vi "GeoData.vi"() -> ()   [LabVIEW 2017] (continued)
TN\tWeakley County\tH1\n38230\t47183\tGreenfield\tTN\tWeakley County\tH1\n38229\t47183\tGleason\tTN\tWeakley County\tH1\n38238\t47183\tMartin\tTN\tWeakley County\tH1\n38261\t47183\tUnion city\tTN\tWeakley County\tH1\n38224\t47183\tCottage grove\tTN\tWeakley County\tH1\n38257\t47183\tSouth fulton\tTN\tWeakley County\tH1\n38241\t47183\tPalmersville\tTN\tWeakley County\tH1\n38506\t47185\tCookeville\tTN\tWhite County\tH1\n38583\t47185\tSparta\tTN\tWhite County\tH1\n38579\t47185\tQuebeck\tTN\tWhite County\tH1\n38587\t47185\tWalling\tTN\tWhite County\tH1\n38559\t47185\tDoyle\tTN\tWhite County\tH1\n37060\t47187\tEagleville\tTN\tWilliamson County\tH1\n37211\t47187\tNashville\tTN\tWilliamson County\tH1\n37179\t47187\tThompsons station\tTN\tWilliamson County\tH1\n37062\t47187\tFairview\tTN\tWilliamson County\tH1\n37215\t47187\tNashville\tTN\tWilliamson County\tH1\n37221\t47187\tNashville\tTN\tWilliamson County\tH1\n37014\t47187\tArrington\tTN\tWilliamson County\tH1\n37174\t47187\tSpring hill\tTN\tWilliamson County\tH1\n37135\t47187\tNolensville\tTN\tWilliamson County\tH1\n37027\t47187\tBrentwood\tTN\tWilliamson County\tH1\n37067\t47187\tFranklin\tTN\tWilliamson County\tH1\n37082\t47187\tKingston springs\tTN\tWilliamson County\tH1\n37046\t47187\tCollege grove\tTN\tWilliamson County\tH1\n37064\t47187\tFranklin\tTN\tWilliamson County\tH1\n38401\t47187\tColumbia\tTN\tWilliamson County\tH1\n37069\t47187\tFranklin\tTN\tWilliamson County\tH1\n37065\t47187\tFranklin\tTN\tWilliamson County\tH1\n38476\t47187\tPrimm springs\tTN\tWilliamson County\tH1\n37025\t47187\tBon aqua\tTN\tWilliamson County\tH1\n37068\t47187\tFranklin\tTN\tWilliamson County\tH1\n37118\t47189\tMilton\tTN\tWilson County\tH1\n37076\t47189\tHermitage\tTN\tWilson County\tH1\n37016\t47189\tAuburntown\tTN\tWilson County\tH1\n37090\t47189\tLebanon\tTN\tWilson County\tH1\n37122\t47189\tMount juliet\tTN\tWilson County\tH1\n37138\t47189\tOld hickory\tTN\tWilson County\tH1\n37095\t47189\tLiberty\tTN\tWilson County\tH1\n37121\t47189\tMount juliet\tTN\tWilson County\tH1\n37012\t47189\tAlexandria\tTN\tWilson County\tH1\n37184\t47189\tWatertown\tTN\tWilson County\tH1\n37088\t47189\tLebanon\tTN\tWilson County\tH1\n37087\t47189\tLebanon\tTN\tWilson County\tH1\n37085\t47189\tLascassas\tTN\tWilson County\tH1\n37071\t47189\tGladeville\tTN\tWilson County\tH1\n75779\t48001\tNeches\tTX\tAnderson County\tH1\n75803\t48001\tPalestine\tTX\tAnderson County\tH1\n75763\t48001\tFrankston\tTX\tAnderson County\tH1\n75844\t48001\tGrapeland\tTX\tAnderson County\tH1\n75751\t48001\tAthens\tTX\tAnderson County\tH1\n75884\t48001\tTennessee colony\tTX\tAnderson County\tH1\n75853\t48001\tMontalba\tTX\tAnderson County\tH1\n75832\t48001\tCayuga\tTX\tAnderson County\tH1\n75861\t48001\tTennessee colony\tTX\tAnderson County\tH1\n75882\t48001\tPalestine\tTX\tAnderson County\tH1\n75839\t48001\tElkhart\tTX\tAnderson County\tH1\n75880\t48001\tTennessee colony\tTX\tAnderson County\tH1\n75801\t48001\tPalestine\tTX\tAnderson County\tH1\n75752\t48001\tAthens\tTX\tAnderson County\tH1\n75770\t48001\tLarue\tTX\tAnderson County\tH1\n75802\t48001\tPalestine\tTX\tAnderson County\tH1\n75886\t48001\tTennessee colony\tTX\tAnderson County\tH1\n79714\t48003\tAndrews\tTX\tAndrews County\tH1\n75915\t48005\tLufkin\tTX\tAngelina County\tH1\n75901\t48005\tLufkin\tTX\tAngelina County\tH1\n75902\t48005\tLufkin\tTX\tAngelina County\tH1\n75949\t48005\tHuntington\tTX\tAngelina County\tH1\n75951\t48005\tJasper\tTX\tAngelina County\tH1\n75980\t48005\tZavalla\tTX\tAngelina County\tH1\n75941\t48005\tDiboll\tTX\tAngelina County\tH1\n75903\t48005\tLufkin\tTX\tAngelina County\tH1\n75904\t48005\tLufkin\tTX\tAngelina County\tH1\n75969\t48005\tPollok\tTX\tAngelina County\tH1\n78382\t48007\tRockport\tTX\tAransas County\tH1\n78390\t48007\tTaft\tTX\tAransas County\tH1\n78381\t48007\tRockport\tTX\tAransas County\tH1\n78336\t48007\tAransas pass\tTX\tAransas County\tH1\n78358\t48007\tFulton\tTX\tAransas County\tH1\n76360\t48009\tElectra\tTX\tArcher County\tH1\n76310\t48009\tWichita falls\tTX\tArcher County\tH1\n76302\t48009\tWichita falls\tTX\tArcher County\tH1\n76374\t48009\tOlney\tTX\tArcher County\tH1\n76366\t48009\tHolliday\tTX\tArcher County\tH1\n76379\t48009\tScotland\tTX\tArcher County\tH1\n76389\t48009\tWindthorst\tTX\tArcher County\tH1\n76370\t48009\tMegargel\tTX\tArcher County\tH1\n76308\t48009\tWichita falls\tTX\tArcher County\tH1\n76351\t48009\tArcher city\tTX\tArcher County\tH1\n79226\t48011\tClarendon\tTX\tArmstrong County\tH1\n79039\t48011\tGroom\tTX\tArmstrong County\tH1\n79042\t48011\tHappy\tTX\tArmstrong County\tH1\n79118\t48011\tAmarillo\tTX\tArmstrong County\tH1\n79019\t48011\tClaude\tTX\tArmstrong County\tH1\n79094\t48011\tWayside\tTX\tArmstrong County\tH1\n78113\t48013\tFalls city\tTX\tAtascosa County\tH1\n78011\t48013\tCharlotte\tTX\tAtascosa County\tH1\n78012\t48013\tChristine\tTX\tAtascosa County\tH1\n78114\t48013\tFloresville\tTX\tAtascosa County\tH1\n78064\t48013\tPleasanton\tTX\tAtascosa County\tH1\n78118\t48013\tKarnes city\tTX\tAtascosa County\tH1\n78052\t48013\tLytle\tTX\tAtascosa County\tH1\n78002\t48013\tAtascosa\tTX\tAtascosa County\tH1\n78065\t48013\tPoteet\tTX\tAtascosa County\tH1\n78264\t48013\tSan antonio\tTX\tAtascosa County\tH1\n78069\t48013\tSomerset\tTX\tAtascosa County\tH1\n78050\t48013\tLeming\tTX\tAtascosa County\tH1\n78073\t48013\tVon ormy\tTX\tAtascosa County\tH1\n78008\t48013\tCampbellton\tTX\tAtascosa County\tH1\n78005\t48013\tBigfoot\tTX\tAtascosa County\tH1\n78021\t48013\tFowlerton\tTX\tAtascosa County\tH1\n78026\t48013\tJourdanton\tTX\tAtascosa County\tH1\n77833\t48015\tBrenham\tTX\tAustin County\tH1\n78933\t48015\tCat spring\tTX\tAustin County\tH1\n77474\t48015\tSealy\tTX\tAustin County\tH1\n78940\t48015\tFayetteville\tTX\tAustin County\tH1\n77452\t48015\tKenney\tTX\tAustin County\tH1\n77835\t48015\tBurton\tTX\tAustin County\tH1\n78954\t48015\tRound top\tTX\tAustin County\tH1\n77418\t48015\tBellville\tTX\tAustin County\tH1\n78944\t48015\tIndustry\tTX\tAustin County\tH1\n77473\t48015\tSan felipe\tTX\tAustin County\tH1\n78950\t48015\tNew ulm\tTX\tAustin County\tH1\n77426\t48015\tChappell hill\tTX\tAustin County\tH1\n77485\t48015\tWallis\tTX\tAustin County\tH1\n78931\t48015\tBleiblerville\tTX\tAustin County\tH1\n79324\t48017\tEnochs\tTX\tBailey County\tH1\n79031\t48017\tEarth\tTX\tBailey County\tH1\n79325\t48017\tFarwell\tTX\tBailey County\tH1\n79346\t48017\tMorton\tTX\tBailey County\tH1\n79347\t48017\tMuleshoe\tTX\tBailey County\tH1\n79344\t48017\tMaple\tTX\tBailey County\tH1\n79371\t48017\tSudan\tTX\tBailey County\tH1\n78023\t48019\tHelotes\tTX\tBandera County\tH1\n78055\t48019\tMedina\tTX\tBandera County\tH1\n78010\t48019\tCenter point\tTX\tBandera County\tH1\n78883\t48019\tTarpley\tTX\tBandera County\tH1\n78063\t48019\tPipe creek\tTX\tBandera County\tH1\n78884\t48019\tUtopia\tTX\tBandera County\tH1\n78003\t48019\tBandera\tTX\tBandera County\tH1\n78885\t48019\tVanderpool\tTX\tBandera County\tH1\n78942\t48021\tGiddings\tTX\tBastrop County\tH1\n78959\t48021\tWaelder\tTX\tBastrop County\tH1\n78616\t48021\tDale\tTX\tBastrop County\tH1\n78659\t48021\tPaige\tTX\tBastrop County\tH1\n78612\t48021\tCedar creek\tTX\tBastrop County\tH1\n78941\t48021\tFlatonia\tTX\tBastrop County\tH1\n78953\t48021\tRosanky\tTX\tBastrop County\tH1\n78617\t48021\tDel valle\tTX\tBastrop County\tH1\n78957\t48021\tSmithville\tTX\tBastrop County\tH1\n78650\t48021\tMc dade\tTX\tBastrop County\tH1\n78662\t48021\tRed rock\tTX\tBastrop County\tH1\n78602\t48021\tBastrop\tTX\tBastrop County\tH1\n78621\t48021\tElgin\tTX\tBastrop County\tH1\n78653\t48021\tManor\tTX\tBastrop County\tH1\n76380\t48023\tSeymour\tTX\tBaylor County\tH1\n78391\t48025\tTynan\tTX\tBee County\tH1\n78162\t48025\tTuleta\tTX\tBee County\tH1\n78102\t48025\tBeeville\tTX\tBee County\tH1\n78119\t48025\tKenedy\tTX\tBee County\tH1\n78389\t48025\tSkidmore\tTX\tBee County\tH1\n78071\t48025\tThree rivers\tTX\tBee County\tH1\n78368\t48025\tMathis\tTX\tBee County\tH1\n78125\t48025\tMineral\tTX\tBee County\tH1\n78142\t48025\tNormanna\tTX\tBee County\tH1\n78145\t48025\tPawnee\tTX\tBee County\tH1\n78104\t48025\tBeeville\tTX\tBee County\tH1\n78146\t48025\tPettus\tTX\tBee County\tH1\n78387\t48025\tSinton\tTX\tBee County\tH1\n76541\t48027\tKilleen\tTX\tBell County\tH1\n76569\t48027\tRogers\tTX\tBell County\tH1\n76519\t48027\tBurlington\tTX\tBell County\tH1\n76533\t48027\tHeidenheimer\tTX\tBell County\tH1\n76502\t48027\tTemple\tTX\tBell County\tH1\n76513\t48027\tBelton\tTX\tBell County\tH1\n76579\t48027\tTroy\tTX\tBell County\tH1\n76528\t48027\tGatesville\tTX\tBell County\tH1\n76557\t48027\tMoody\tTX\tBell County\tH1\n76559\t48027\tNolanville\tTX\tBell County\tH1\n76537\t48027\tJarrell\tTX\tBell County\tH1\n76547\t48027\tKilleen\tTX\tBell County\tH1\n76549\t48027\tKilleen\tTX\tBell County\tH1\n76508\t48027\tTemple\tTX\tBell County\tH1\n76542\t48027\tKilleen\tTX\tBell County\tH1\n76548\t48027\tHarker heights\tTX\tBell County\tH1\n76571\t48027\tSalado\tTX\tBell County\tH1\n76527\t48027\tFlorence\tTX\tBell County\tH1\n76570\t48027\tRosebud\tTX\tBell County\tH1\n76504\t48027\tTemple\tTX\tBell County\tH1\n76554\t48027\tLittle river academy\tTX\tBell County\tH1\n76539\t48027\tKempner\tTX\tBell County\tH1\n76540\t48027\tKilleen\tTX\tBell County\tH1\n76501\t48027\tTemple\tTX\tBell County\tH1\n76564\t48027\tPendleton\tTX\tBell County\tH1\n76503\t48027\tTemple\tTX\tBell County\tH1\n76543\t48027\tKilleen\tTX\tBell County\tH1\n76511\t48027\tBartlett\tTX\tBell County\tH1\n76544\t48027\tFort hood\tTX\tBell County\tH1\n76656\t48027\tLott\tTX\tBell County\tH1\n76534\t48027\tHolland\tTX\tBell County\tH1\n78023\t48029\tHelotes\tTX\tBexar County\tH1\n78039\t48029\tLa coste\tTX\tBexar County\tH1\n78210\t48029\tSan antonio\tTX\tBexar County\tH1\n78260\t48029\tSan antonio\tTX\tBexar County\tH1\n78270\t48029\tSan antonio\tTX\tBexar County\tH1\n78239\t48029\tSan antonio\tTX\tBexar County\tH1\n78244\t48029\tSan antonio\tTX\tBexar County\tH1\n78235\t48029\tSan antonio\tTX\tBexar County\tH1\n78288\t48029\tSan antonio\tTX\tBexar County\tH1\n78297\t48029\tSan antonio\tTX\tBexar County\tH1\n78246\t48029\tSan antonio\tTX\tBexar County\tH1\n78124\t48029\tMarion\tTX\tBexar County\tH1\n78214\t48029\tSan antonio\tTX\tBexar County\tH1\n78202\t48029\tSan antonio\tTX\tBexar County\tH1\n78207\t48029\tSan antonio\tTX\tBexar County\tH1\n78222\t48029\tSan antonio\tTX\tBexar County\tH1\n78224\t48029\tSan antonio\tTX\tBexar County\tH1\n78259\t48029\tSan antonio\tTX\tBexar County\tH1\n78150\t48029\tJbsa randolph\tTX\tBexar County\tH1\n78296\t48029\tSan antonio\tTX\tBexar County\tH1\n78291\t48029\tSan antonio\tTX\tBexar County\tH1\n78054\t48029\tMacdona\tTX\tBexar County\tH1\n78148\t48029\tUniversal city\tTX\tBexar County\tH1\n78217\t48029\tSan antonio\tTX\tBexar County\tH1\n78208\t48029\tSan antonio\tTX\tBexar County\tH1\n78215\t48029\tSan antonio\tTX\tBexar County\tH1\n78225\t48029\tSan antonio\tTX\tBexar County\tH1\n78226\t48029\tSan antonio\tTX\tBexar County\tH1\n78250\t48029\tSan antonio\tTX\tBexar County\tH1\n78266\t48029\tSan antonio\tTX\tBexar County\tH1\n78263\t48029\tSan antonio\tTX\tBexar County\tH1\n78206\t48029\tSan antonio\tTX\tBexar County\tH1\n78268\t48029\tSan antonio\tTX\tBexar County\tH1\n78298\t48029\tSan antonio\tTX\tBexar County\tH1\n78294\t48029\tSan antonio\tTX\tBexar County\tH1\n78292\t48029\tSan antonio\tTX\tBexar County\tH1\n78006\t48029\tBoerne\tTX\tBexar County\tH1\n78108\t48029\tCibolo\tTX\tBexar County\tH1\n78052\t48029\tLytle\tTX\tBexar County\tH1\n78212\t48029\tSan antonio\tTX\tBexar County\tH1\n78205\t48029\tSan antonio\tTX\tBexar County\tH1\n78229\t48029\tSan antonio\tTX\tBexar County\tH1\n78233\t48029\tSan antonio\tTX\tBexar County\tH1\n78232\t48029\tSan antonio\tTX\tBexar County\tH1\n78240\t48029\tSan antonio\tTX\tBexar County\tH1\n78237\t48029\tSan antonio\tTX\tBexar County\tH1\n78251\t48029\tSan antonio\tTX\tBexar County\tH1\n78269\t48029\tSan antonio\tTX\tBexar County\tH1\n78002\t48029\tAtascosa\tTX\tBexar County\tH1\n78101\t48029\tAdkins\tTX\tBexar County\tH1\n78209\t48029\tSan antonio\tTX\tBexar County\tH1\n78220\t48029\tSan antonio\tTX\tBexar County\tH1\n78216\t48029\tSan antonio\tTX\tBexar County\tH1\n78163\t48029\tBulverde\tTX\tBexar County\tH1\n78204\t48029\tSan antonio\tTX\tBexar County\tH1\n78231\t48029\tSan antonio\tTX\tBexar County\tH1\n78264\t48029\tSan antonio\tTX\tBexar County\tH1\n78256\t48029\tSan antonio\tTX\tBexar County\tH1\n78234\t48029\tJbsa ft sam houston\tTX\tBexar County\tH1\n78253\t48029\tSan antonio\tTX\tBexar County\tH1\n78254\t48029\tSan antonio\tTX\tBexar County\tH1\n78069\t48029\tSomerset\tTX\tBexar County\tH1\n78299\t48029\tSan antonio\tTX\tBexar County\tH1\n78252\t48029\tSan antonio\tTX\tBexar County\tH1\n78284\t48029\tSan antonio\tTX\tBexar County\tH1\n78285\t48029\tSan antonio\tTX\tBexar County\tH1\n78009\t48029\tCastroville\tTX\tBexar County\tH1\n78073\t48029\tVon ormy\tTX\tBexar County\tH1\n78154\t48029\tSchertz\tTX\tBexar County\tH1\n78221\t48029\tSan antonio\tTX\tBexar County\tH1\n78201\t48029\tSan antonio\tTX\tBexar County\tH1\n78213\t48029\tSan antonio\tTX\tBexar County\tH1\n78228\t48029\tSan antonio\tTX\tBexar County\tH1\n78230\t48029\tSan antonio\tTX\tBexar County\tH1\n78258\t48029\tSan antonio\tTX\tBexar County\tH1\n78245\t48029\tSan antonio\tTX\tBexar County\tH1\n78242\t48029\tSan antonio\tTX\tBexar County\tH1\n78238\t48029\tSan antonio\tTX\tBexar County\tH1\n78295\t48029\tSan antonio\tTX\tBexar County\tH1\n78152\t48029\tSaint hedwig\tTX\tBexar County\tH1\n78243\t48029\tSan antonio\tTX\tBexar County\tH1\n78015\t48029\tBoerne\tTX\tBexar County\tH1\n78109\t48029\tConverse\tTX\tBexar County\tH1\n78112\t48029\tElmendorf\tTX\tBexar County\tH1\n78218\t48029\tSan antonio\tTX\tBexar County\tH1\n78219\t48029\tSan antonio\tTX\tBexar County\tH1\n78223\t48029\tSan antonio\tTX\tBexar County\tH1\n78227\t48029\tSan antonio\tTX\tBexar County\tH1\n78203\t48029\tSan antonio\tTX\tBexar County\tH1\n78247\t48029\tSan antonio\tTX\tBexar County\tH1\n78249\t48029\tSan antonio\tTX\tBexar County\tH1\n78257\t48029\tSan antonio\tTX\tBexar County\tH1\n78283\t48029\tSan antonio\tTX\tBexar County\tH1\n78265\t48029\tSan antonio\tTX\tBexar County\tH1\n78278\t48029\tSan antonio\tTX\tBexar County\tH1\n78293\t48029\tSan antonio\tTX\tBexar County\tH1\n78241\t48029\tSan antonio\tTX\tBexar County\tH1\n78211\t48029\tSan antonio\tTX\tBexar County\tH1\n78248\t48029\tSan antonio\tTX\tBexar County\tH1\n78236\t48029\tJbsa lackland\tTX\tBexar County\tH1\n78255\t48029\tSan antonio\tTX\tBexar County\tH1\n78261\t48029\tSan antonio\tTX\tBexar County\tH1\n78280\t48029\tSan antonio\tTX\tBexar County\tH1\n78279\t48029\tSan antonio\tTX\tBexar County\tH1\n78635\t48031\tHye\tTX\tBlanco County\tH1\n78027\t48031\tKendalia\tTX\tBlanco County\tH1\n78620\t48031\tDripping springs\tTX\tBlanco County\tH1\n78636\t48031\tJohnson city\tTX\tBlanco County\tH1\n78663\t48031\tRound mountain\tTX\tBlanco County\tH1\n78676\t48031\tWimberley\tTX\tBlanco County\tH1\n78070\t48031\tSpring branch\tTX\tBlanco County\tH1\n78669\t48031\tSpicewood\tTX\tBlanco County\tH1\n78671\t48031\tStonewall\tTX\tBlanco County\tH1\n78606\t48031\tBlanco\tTX\tBlanco County\tH1\n79356\t48033\tPost\tTX\tBorden County\tH1\n79713\t48033\tAckerly\tTX\tBorden County\tH1\n79738\t48033\tGail\tTX\tBorden County\tH1\n79511\t48033\tCoahoma\tTX\tBorden County\tH1\n79517\t48033\tFluvanna\tTX\tBorden County\tH1\n79527\t48033\tIra\tTX\tBorden County\tH1\n79351\t48033\tOdonnell\tTX\tBorden County\tH1\n76633\t48035\tChina spring\tTX\tBosque County\tH1\n76043\t48035\tGlen rose\tTX\tBosque County\tH1\n76528\t48035\tGatesville\tTX\tBosque County\tH1\n76652\t48035\tKopperl\tTX\tBosque County\tH1\n76457\t48035\tHico\tTX\tBosque County\tH1\n76634\t48035\tClifton\tTX\tBosque County\tH1\n76665\t48035\tMeridian\tTX\tBosque County\tH1\n76671\t48035\tMorgan\tTX\tBosque County\tH1\n76649\t48035\tIredell\tTX\tBosque County\tH1\n76689\t48035\tValley mills\tTX\tBosque County\tH1\n76690\t48035\tWalnut springs\tTX\tBosque County\tH1\n76637\t48035\tCranfills gap\tTX\tBosque County\tH1\n75501\t48037\tTexarkana\tTX\tBowie County\tH1\n75560\t48037\tDouglassville\tTX\tBowie County\tH1\n75573\t48037\tRedwater\tTX\tBowie County\tH1\n75567\t48037\tMaud\tTX\tBowie County\tH1\n75554\t48037\tAvery\tTX\tBowie County\tH1\n75503\t48037\tTexarkana\tTX\tBowie County\tH1\n75505\t48037\tTexarkana\tTX\tBowie County\tH1\n75570\t48037\tNew boston\tTX\tBowie County\tH1\n75561\t48037\tHooks\tTX\tBowie County\tH1\n75504\t48037\tTexarkana\tTX\tBowie County\tH1\n75599\t48037\tTexarkana\tTX\tBowie County\tH1\n75559\t48037\tDe kalb\tTX\tBowie County\tH1\n75574\t48037\tSimms\tTX\tBowie County\tH1\n75569\t48037\tNash\tTX\tBowie County\tH1\n77422\t48039\tBrazoria\tTX\tBrazoria County\tH1\n77510\t48039\tSanta fe\tTX\tBrazoria County\tH1\n77541\t48039\tFreeport\tTX\tBrazoria County\tH1\n77566\t48039\tLake jackson\tTX\tBrazoria County\tH1\n77584\t48039\tPearland\tTX\tBrazoria County\tH1\n77515\t48039\tAngleton\tTX\tBrazoria County\tH1\n77517\t48039\tSanta fe\tTX\tBrazoria County\tH1\n77546\t48039\tFriendswood\tTX\tBrazoria County\tH1\n77542\t48039\tFreeport\tTX\tBrazoria County\tH1\n77583\t48039\tRosharon\tTX\tBrazoria County\tH1\n77581\t48039\tPearland\tTX\tBrazoria County\tH1\n77588\t48039\tPearland\tTX\tBrazoria County\tH1\n77430\t48039\tDamon\tTX\tBrazoria County\tH1\n77486\t48039\tWest columbia\tTX\tBrazoria County\tH1\n77444\t48039\tGuy\tTX\tBrazoria County\tH1\n77516\t48039\tAngleton\tTX\tBrazoria County\tH1\n77463\t48039\tOld ocean\tTX\tBrazoria County\tH1\n77431\t48039\tDanciger\tTX\tBrazoria County\tH1\n77480\t48039\tSweeny\tTX\tBrazoria County\tH1\n77531\t48039\tClute\tTX\tBrazoria County\tH1\n77545\t48039\tFresno\tTX\tBrazoria County\tH1\n77578\t48039\tManvel\tTX\tBrazoria County\tH1\n77534\t48039\tDanbury\tTX\tBrazoria County\tH1\n77511\t48039\tAlvin\tTX\tBrazoria County\tH1\n77512\t48039\tAlvin\tTX\tBrazoria County\tH1\n77577\t48039\tLiverpool\tTX\tBrazoria County\tH1\n77840\t48041\tCollege station\tTX\tBrazos County\tH1\n77805\t48041\tBryan\tTX\tBrazos County\tH1\n77843\t48041\tCollege station\tTX\tBrazos County\tH1\n77806\t48041\tBryan\tTX\tBrazos County\tH1\n77868\t48041\tNavasota\tTX\tBrazos County\tH1\n77856\t48041\tFranklin\tTX\tBrazos County\tH1\n77859\t48041\tHearne\tTX\tBrazos County\tH1\n77841\t48041\tCollege station\tTX\tBrazos County\tH1\n77807\t48041\tBryan\tTX\tBrazos County\tH1\n77844\t48041\tCollege station\tTX\tBrazos County\tH1\n77866\t48041\tMillican\tTX\tBrazos County\tH1\n77801\t48041\tBryan\tTX\tBrazos County\tH1\n77842\t48041\tCollege station\tTX\tBrazos County\tH1\n77808\t48041\tBryan\tTX\tBrazos County\tH1\n77802\t48041\tBryan\tTX\tBrazos County\tH1\n77881\t48041\tWellborn\tTX\tBrazos County\tH1\n77862\t48041\tKurten\tTX\tBrazos County\tH1\n77845\t48041\tCollege station\tTX\tBrazos County\tH1\n77803\t48041\tBryan\tTX\tBrazos County\tH1\n79830\t48043\tAlpine\tTX\tBrewster County\tH1\n79834\t48043\tBig bend national park\tTX\tBrewster County\tH1\n79832\t48043\tAlpine\tTX\tBrewster County\tH1\n79852\t48043\tTerlingua\tTX\tBrewster County\tH1\n79842\t48043\tMarathon\tTX\tBrewster County\tH1\n79257\t48045\tSilverton\tTX\tBriscoe County\tH1\n79261\t48045\tTurkey\tTX\tBriscoe County\tH1\n79255\t48045\tQuitaque\tTX\tBriscoe County\tH1\n78353\t48047\tEncino\tTX\tBrooks County\tH1\n78355\t48047\tFalfurrias\tTX\tBrooks County\tH1\n76823\t48049\tBangs\tTX\tBrown County\tH1\n76857\t48049\tMay\tTX\tBrown County\tH1\n76827\t48049\tBrookesmith\tTX\tBrown County\tH1\n76471\t48049\tRising star\tTX\tBrown County\tH1\n76890\t48049\tZephyr\tTX\tBrown County\tH1\n76804\t48049\tBrownwood\tTX\tBrown County\tH1\n76878\t48049\tSanta anna\tTX\tBrown County\tH1\n76803\t48049\tEarly\tTX\tBrown County\tH1\n76802\t48049\tEarly\tTX\tBrown County\tH1\n76443\t48049\tCross plains\tTX\tBrown County\tH1\n76801\t48049\tBrownwood\tTX\tBrown County\tH1\n76432\t48049\tBlanket\tTX\tBrown County\tH1\n77878\t48051\tSnook\tTX\tBurleson County\tH1\n77838\t48051\tChriesman\tTX\tBurleson County\tH1\n77879\t48051\tSomerville\tTX\tBurleson County\tH1\n77836\t48051\tCaldwell\tTX\tBurleson County\tH1\n77852\t48051\tDeanville\tTX\tBurleson County\tH1\n77863\t48051\tLyons\tTX\tBurleson County\tH1\n76550\t48053\tLampasas\tTX\tBurnet County\tH1\n78605\t48053\tBertram\tTX\tBurnet County\tH1\n76549\t48053\tKilleen\tTX\tBurnet County\tH1\n78639\t48053\tKingsland\tTX\tBurnet County\tH1\n76527\t48053\tFlorence\tTX\tBurnet County\tH1\n78642\t48053\tLiberty hill\tTX\tBurnet County\tH1\n78611\t48053\tBurnet\tTX\tBurnet County\tH1\n76539\t48053\tKempner\tTX\tBurnet County\tH1\n78654\t48053\tMarble falls\tTX\tBurnet County\tH1\n78663\t48053\tRound mountain\tTX\tBurnet County\tH1\n78657\t48053\tHorseshoe bay\tTX\tBurnet County\tH1\n78608\t48053\tBriggs\tTX\tBurnet County\tH1\n78669\t48053\tSpicewood\tTX\tBurnet County\tH1\n78959\t48055\tWaelder\tTX\tCaldwell County\tH1\n78632\t48055\tHarwood\tTX\tCaldwell County\tH1\n78616\t48055\tDale\tTX\tCaldwell County\tH1\n78953\t48055\tRosanky\tTX\tCaldwell County\tH1\n78666\t48055\tSan marcos\tTX\tCaldwell County\tH1\n78644\t48055\tLockhart\tTX\tCaldwell County\tH1\n78640\t48055\tKyle\tTX\tCaldwell County\tH1\n78610\t48055\tBuda\tTX\tCaldwell County\tH1\n78656\t48055\tMaxwell\tTX\tCaldwell County\tH1\n78661\t48055\tPrairie lea\tTX\tCaldwell County\tH1\n78662\t48055\tRed rock\tTX\tCaldwell County\tH1\n78648\t48055\tLuling\tTX\tCaldwell County\tH1\n78622\t48055\tFentress\tTX\tCaldwell County\tH1\n78655\t48055\tMartindale\tTX\tCaldwell County\tH1\n77979\t48057\tPort lavaca\tTX\tCalhoun County\tH1\n77465\t48057\tPalacios\tTX\tCalhoun County\tH1\n77990\t48057\tTivoli\tTX\tCalhoun County\tH1\n77982\t48057\tPort o connor\tTX\tCalhoun County\tH1\n77983\t48057\tSeadrift\tTX\tCalhoun County\tH1\n77978\t48057\tPoint comfort\tTX\tCalhoun County\tH1\n79504\t48059\tBaird\tTX\tCallahan County\tH1\n79601\t48059\tAbilene\tTX\tCallahan County\tH1\n76437\t48059\tCisco\tTX\tCallahan County\tH1\n76464\t48059\tMoran\tTX\tCallahan County\tH1\n76469\t48059\tPutnam\tTX\tCallahan County\tH1\n76443\t48059\tCross plains\tTX\tCallahan County\tH1\n79602\t48059\tAbilene\tTX\tCallahan County\tH1\n79510\t48059\tClyde\tTX\tCallahan County\tH1\n78569\t48061\tLyford\tTX\tCameron County\tH1\n78535\t48061\tCombes\tTX\tCameron County\tH1\n78592\t48061\tSanta maria\tTX\tCameron County\tH1\n78522\t48061\tBrownsville\tTX\tCameron County\tH1\n78550\t48061\tHarlingen\tTX\tCameron County\tH1\n78552\t48061\tHarlingen\tTX\tCameron County\tH1\n78553\t48061\tHarlingen\tTX\tCameron County\tH1\n78567\t48061\tLos indios\tTX\tCameron County\tH1\n78521\t48061\tBrownsville\tTX\tCameron County\tH1\n78583\t48061\tRio hondo\tTX\tCameron County\tH1\n78597\t48061\tSouth padre island\tTX\tCameron County\tH1\n78586\t48061\tSan benito\tTX\tCameron County\tH1\n78575\t48061\tOlmito\tTX\tCameron County\tH1\n78523\t48061\tBrownsville\tTX\tCameron County\tH1\n78593\t48061\tSanta rosa\tTX\tCameron County\tH1\n78520\t48061\tBrownsville\tTX\tCameron County\tH1\n78570\t48061\tMercedes\tTX\tCameron County\tH1\n78566\t48061\tLos fresnos\tTX\tCameron County\tH1\n78551\t48061\tHarlingen\tTX\tCameron County\tH1\n78559\t48061\tLa feria\tTX\tCameron County\tH1\n78526\t48061\tBrownsville\tTX\tCameron County\tH1\n78578\t48061\tPort isabel\tTX\tCameron County\tH1\n78568\t48061\tLozano\tTX\tCameron County\tH1\n75451\t48063\tLeesburg\tTX\tCamp County\tH1\n75644\t48063\tGilmer\tTX\tCamp County\tH1\n75494\t48063\tWinnsboro\tTX\tCamp County\tH1\n75686\t48063\tPittsburg\tTX\tCamp County\tH1\n79080\t48065\tSkellytown\tTX\tCarson County\tH1\n79068\t48065\tPanhandle\tTX\tCarson County\tH1\n79108\t48065\tAmarillo\tTX\tCarson County\tH1\n79036\t48065\tFritch\tTX\tCarson County\tH1\n79097\t48065\tWhite deer\tTX\tCarson County\tH1\n79039\t48065\tGroom\tTX\tCarson County\tH1\n75572\t48067\tQueen city\tTX\tCass County\tH1\n75560\t48067\tDouglassville\tTX\tCass County\tH1\n75638\t48067\tDaingerfield\tTX\tCass County\tH1\n75630\t48067\tAvinger\tTX\tCass County\tH1\n75551\t48067\tAtlanta\tTX\tCass County\tH1\n75555\t48067\tBivins\tTX\tCass County\tH1\n75556\t48067\tBloomburg\tTX\tCass County\tH1\n75563\t48067\tLinden\tTX\tCass County\tH1\n75568\t48067\tNaples\tTX\tCass County\tH1\n75657\t48067\tJefferson\tTX\tCass County\tH1\n75566\t48067\tMarietta\tTX\tCass County\tH1\n75565\t48067\tMc leod\tTX\tCass County\tH1\n75656\t48067\tHughes springs\tTX\tCass County\tH1\n75562\t48067\tKildare\tTX\tCass County\tH1\n79045\t48069\tHereford\tTX\tCastro County\tH1\n79027\t48069\tDimmitt\tTX\tCastro County\tH1\n79043\t48069\tHart\tTX\tCastro County\tH1\n79031\t48069\tEarth\tTX\tCastro County\tH1\n79035\t48069\tFriona\tTX\tCastro County\tH1\n79347\t48069\tMuleshoe\tTX\tCastro County\tH1\n79063\t48069\tNazareth\tTX\tCastro County\tH1\n79085\t48069\tSummerfield\tTX\tCastro County\tH1\n77597\t48071\tWallisville\tTX\tChambers County\tH1\n77661\t48071\tStowell\tTX\tChambers County\tH1\n77521\t48071\tBaytown\tTX\tChambers County\tH1\n77580\t48071\tMont belvieu\tTX\tChambers County\tH1\n77514\t48071\tAnahuac\tTX\tChambers County\tH1\n77535\t48071\tDayton\tTX\tChambers County\tH1\n77665\t48071\tWinnie\tTX\tChambers County\tH1\n77575\t48071\tLiberty\tTX\tChambers County\tH1\n77560\t48071\tHankamer\tTX\tChambers County\tH1\n77523\t48071\tBaytown\tTX\tChambers County\tH1\n75759\t48073\tCuney\tTX\tCherokee County\tH1\n75764\t48073\tGallatin\tTX\tCherokee County\tH1\n75784\t48073\tReklaw\tTX\tCherokee County\tH1\n75976\t48073\tWells\tTX\tCherokee County\tH1\n75789\t48073\tTroup\tTX\tCherokee County\tH1\n75925\t48073\tAlto\tTX\tCherokee County\tH1\n75766\t48073\tJacksonville\tTX\tCherokee County\tH1\n75772\t48073\tMaydelle\tTX\tCherokee County\tH1\n75785\t48073\tRusk\tTX\tCherokee County\tH1\n75969\t48073\tPollok\tTX\tCherokee County\tH1\n75757\t48073\tBullard\tTX\tCherokee County\tH1\n75780\t48073\tNew summerfield\tTX\tCherokee County\tH1\n79230\t48075\tDodson\tTX\tChildress County\tH1\n79201\t48075\tChildress\tTX\tChildress County\tH1\n79095\t48075\tWellington\tTX\tChildress County\tH1\n79259\t48075\tTell\tTX\tChildress County\tH1\n76305\t48077\tWichita falls\tTX\tClay County\tH1\n76310\t48077\tWichita falls\tTX\tClay County\tH1\n76365\t48077\tHenrietta\tTX\tClay County\tH1\n76357\t48077\tByers\tTX\tClay County\tH1\n76377\t48077\tPetrolia\tTX\tClay County\tH1\n76228\t48077\tBellevue\tTX\tClay County\tH1\n76352\t48077\tBluegrove\tTX\tClay County\tH1\n76230\t48077\tBowie\tTX\tClay County\tH1\n76379\t48077\tScotland\tTX\tClay County\tH1\n76389\t48077\tWindthorst\tTX\tClay County\tH1\n76261\t48077\tRinggold\tTX\tClay County\tH1\n79379\t48079\tWhiteface\tTX\tCochran County\tH1\n79346\t48079\tMorton\tTX\tCochran County\tH1\n79314\t48079\tBledsoe\tTX\tCochran County\tH1\n79336\t48079\tLevelland\tTX\tCochran County\tH1\n76945\t48081\tRobert lee\tTX\tCoke County\tH1\n76905\t48081\tSan angelo\tTX\tCoke County\tH1\n79506\t48081\tBlackwell\tTX\tCoke County\tH1\n76861\t48081\tMiles\tTX\tCoke County\tH1\n76933\t48081\tBronte\tTX\tCoke County\tH1\n76953\t48081\tTennyson\tTX\tCoke County\tH1\n76949\t48081\tSilver\tTX\tCoke County\tH1\n76873\t48083\tRockwood\tTX\tColeman County\tH1\n76823\t48083\tBangs\tTX\tColeman County\tH1\n76845\t48083\tGouldbusk\tTX\tColeman County\tH1\n76884\t48083\tValera\tTX\tColeman County\tH1\n76878\t48083\tSanta anna\tTX\tColeman County\tH1\n76834\t48083\tColeman\tTX\tColeman County\tH1\n79519\t48083\tGoldsboro\tTX\tColeman County\tH1\n79538\t48083\tNovice\tTX\tColeman County\tH1\n76882\t48083\tTalpa\tTX\tColeman County\tH1\n76828\t48083\tBurkett\tTX\tColeman County\tH1\n76443\t48083\tCross plains\tTX\tColeman County\tH1\n79510\t48083\tClyde\tTX\tColeman County\tH1\n76888\t48083\tVoss\tTX\tColeman County\tH1\n75098\t48085\tWylie\tTX\tCollin County\tH1\n75071\t48085\tMckinney\tTX\tCollin County\tH1\n75075\t48085\tPlano\tTX\tCollin County\tH1\n75409\t48085\tAnna\tTX\tCollin County\tH1\n75121\t48085\tCopeville\tTX\tCollin County\tH1\n75485\t48085\tWestminster\tTX\tCollin County\tH1\n75164\t48085\tJosephine\tTX\tCollin County\tH1\n75166\t48085\tLavon\tTX\tCollin County\tH1\n75058\t48085\tGunter\tTX\tCollin County\tH1\n75407\t48085\tPrinceton\tTX\tCollin County\tH1\n75379\t48085\tDallas\tTX\tCollin County\tH1\n75026\t48085\tPlano\tTX\tCollin County\tH1\n75033\t48085\tFrisco\tTX\tCollin County\tH1\n75048\t48085\tSachse\tTX\tCollin County\tH1\n75069\t48085\tMckinney\tTX\tCollin County\tH1\n75074\t48085\tPlano\tTX\tCollin County\tH1\n75070\t48085\tMckinney\tTX\tCollin County\tH1\n75080\t48085\tRichardson\tTX\tCollin County\tH1\n75442\t48085\tFarmersville\tTX\tCollin County\tH1\n75287\t48085\tDallas\tTX\tCollin County\tH1\n75370\t48085\tDallas\tTX\tCollin County\tH1\n75023\t48085\tPlano\tTX\tCollin County\tH1\n75087\t48085\tRockwall\tTX\tCollin County\tH1\n75173\t48085\tNevada\tTX\tCollin County\tH1\n75252\t48085\tDallas\tTX\tCollin County\tH1\n75086\t48085\tPlano\tTX\tCollin County\tH1\n75002\t48085\tAllen\tTX\tCollin County\tH1\n75009\t48085\tCelina\tTX\tCollin County\tH1\n75097\t48085\tWeston\tTX\tCollin County\tH1\n75025\t48085\tPlano\tTX\tCollin County\tH1\n75044\t48085\tGarland\tTX\tCollin County\tH1\n75093\t48085\tPlano\tTX\tCollin County\tH1\n75094\t48085\tPlano\tTX\tCollin County\tH1\n75452\t48085\tLeonard\tTX\tCollin County\tH1\n75007\t48085\tCarrollton\tTX\tCollin County\tH1\n75013\t48085\tAllen\tTX\tCollin County\tH1\n75024\t48085\tPlano\tTX\tCollin County\tH1\n75248\t48085\tDallas\tTX\tCollin County\tH1\n75082\t48085\tRichardson\tTX\tCollin County\tH1\n75454\t48085\tMelissa\tTX\tCollin County\tH1\n75495\t48085\tVan alstyne\tTX\tCollin County\tH1\n75034\t48085\tFrisco\tTX\tCollin County\tH1\n75035\t48085\tFrisco\tTX\tCollin County\tH1\n75189\t48085\tRoyse city\tTX\tCollin County\tH1\n75078\t48085\tProsper\tTX\tCollin County\tH1\n75424\t48085\tBlue ridge\tTX\tCollin County\tH1\n75491\t48085\tWhitewright\tTX\tCollin County\tH1\n79079\t48087\tShamrock\tTX\tCollingsworth County\tH1\n79230\t48087\tDodson\tTX\tCollingsworth County\tH1\n79251\t48087\tQuail\tTX\tCollingsworth County\tH1\n79245\t48087\tMemphis\tTX\tCollingsworth County\tH1\n79095\t48087\tWellington\tTX\tCollingsworth County\tH1\n78933\t48089\tCat spring\tTX\tColorado County\tH1\n78934\t48089\tColumbus\tTX\tColorado County\tH1\n77475\t48089\tSheridan\tTX\tColorado County\tH1\n77474\t48089\tSealy\tTX\tColorado County\tH1\n78951\t48089\tOakland\tTX\tColorado County\tH1\n78943\t48089\tGlidden\tTX\tColorado County\tH1\n78940\t48089\tFayetteville\tTX\tColorado County\tH1\n78956\t48089\tSchulenburg\tTX\tColorado County\tH1\n77435\t48089\tEast bernard\tTX\tColorado County\tH1\n77442\t48089\tGarwood\tTX\tColorado County\tH1\n78935\t48089\tAlleyton\tTX\tColorado County\tH1\n78962\t48089\tWeimar\tTX\tColorado County\tH1\n77434\t48089\tEagle lake\tTX\tColorado County\tH1\n78950\t48089\tNew ulm\tTX\tColorado County\tH1\n77470\t48089\tRock island\tTX\tColorado County\tH1\n77964\t48089\tHallettsville\tTX\tColorado County\tH1\n77460\t48089\tNada\tTX\tColorado County\tH1\n77412\t48089\tAltair\tTX\tColorado County\tH1\n78132\t48091\tNew braunfels\tTX\tComal County\tH1\n78131\t48091\tNew braunfels\tTX\tComal County\tH1\n78130\t48091\tNew braunfels\tTX\tComal County\tH1\n78266\t48091\tSan antonio\tTX\tComal County\tH1\n78006\t48091\tBoerne\tTX\tComal County\tH1\n78108\t48091\tCibolo\tTX\tComal County\tH1\n78666\t48091\tSan marcos\tTX\tComal County\tH1\n78133\t48091\tCanyon lake\tTX\tComal County\tH1\n78163\t48091\tBulverde\tTX\tComal County\tH1\n78623\t48091\tFischer\tTX\tComal County\tH1\n78154\t48091\tSchertz\tTX\tComal County\tH1\n78676\t48091\tWimberley\tTX\tComal County\tH1\n78135\t48091\tNew braunfels\tTX\tComal County\tH1\n78015\t48091\tBoerne\tTX\tComal County\tH1\n78070\t48091\tSpring branch\tTX\tComal County\tH1\n78606\t48091\tBlanco\tTX\tComal County\tH1\n76436\t48093\tCarlton\tTX\tComanche County\tH1\n76468\t48093\tProctor\tTX\tComanche County\tH1\n76471\t48093\tRising star\tTX\tComanche County\tH1\n76890\t48093\tZephyr\tTX\tComanche County\tH1\n76442\t48093\tComanche\tTX\tComanche County\tH1\n76446\t48093\tDublin\tTX\tComanche County\tH1\n76474\t48093\tSidney\tTX\tComanche County\tH1\n76444\t48093\tDe leon\tTX\tComanche County\tH1\n76445\t48093\tDesdemona\tTX\tComanche County\tH1\n76455\t48093\tGustine\tTX\tComanche County\tH1\n76452\t48093\tEnergy\tTX\tComanche County\tH1\n76454\t48093\tGorman\tTX\tComanche County\tH1\n76432\t48093\tBlanket\tTX\tComanche County\tH1\n76855\t48095\tLowake\tTX\tConcho County\tH1\n76862\t48095\tMillersview\tTX\tConcho County\tH1\n76866\t48095\tPaint rock\tTX\tConcho County\tH1\n76861\t48095\tMiles\tTX\tConcho County\tH1\n76875\t48095\tRowena\tTX\tConcho County\tH1\n76858\t48095\tMelvin\tTX\tConcho County\tH1\n76940\t48095\tMereta\tTX\tConcho County\tH1\n76937\t48095\tEola\tTX\tConcho County\tH1\n76837\t48095\tEden\tTX\tConcho County\tH1\n76252\t48097\tMuenster\tTX\tCooke County\tH1\n76258\t48097\tPilot point\tTX\tCooke County\tH1\n76233\t48097\tCollinsville\tTX\tCooke County\tH1\n76240\t48097\tGainesville\tTX\tCooke County\tH1\n76265\t48097\tSaint jo\tTX\tCooke County\tH1\n76271\t48097\tTioga\tTX\tCooke County\tH1\n76253\t48097\tMyra\tTX\tCooke County\tH1\n76234\t48097\tDecatur\tTX\tCooke County\tH1\n76241\t48097\tGainesville\tTX\tCooke County\tH1\n76250\t48097\tLindsay\tTX\tCooke County\tH1\n76266\t48097\tSanger\tTX\tCooke County\tH1\n76273\t48097\tWhitesboro\tTX\tCooke County\tH1\n76263\t48097\tRosston\tTX\tCooke County\tH1\n76239\t48097\tForestburg\tTX\tCooke County\tH1\n76238\t48097\tEra\tTX\tCooke County\tH1\n76272\t48097\tValley view\tTX\tCooke County\tH1\n76528\t48099\tGatesville\tTX\tCoryell County\tH1\n76557\t48099\tMoody\tTX\tCoryell County\tH1\n76558\t48099\tMound\tTX\tCoryell County\tH1\n76549\t48099\tKilleen\tTX\tCoryell County\tH1\n76634\t48099\tClifton\tTX\tCoryell County\tH1\n76689\t48099\tValley mills\tTX\tCoryell County\tH1\n76538\t48099\tJonesboro\tTX\tCoryell County\tH1\n76539\t48099\tKempner\tTX\tCoryell County\tH1\n76657\t48099\tMc gregor\tTX\tCoryell County\tH1\n76638\t48099\tCrawford\tTX\tCoryell County\tH1\n76598\t48099\tGatesville\tTX\tCoryell County\tH1\n76525\t48099\tEvant\tTX\tCoryell County\tH1\n76561\t48099\tOglesby\tTX\tCoryell County\tH1\n76599\t48099\tGatesville\tTX\tCoryell County\tH1\n76526\t48099\tFlat\tTX\tCoryell County\tH1\n76522\t48099\tCopperas cove\tTX\tCoryell County\tH1\n76596\t48099\tGatesville\tTX\tCoryell County\tH1\n76544\t48099\tFort hood\tTX\tCoryell County\tH1\n76566\t48099\tPurmela\tTX\tCoryell County\tH1\n76597\t48099\tGatesville\tTX\tCoryell County\tH1\n79223\t48101\tCee vee\tTX\tCottle County\tH1\n79248\t48101\tPaducah\tTX\tCottle County\tH1\n79731\t48103\tCrane\tTX\tCrane County\tH1\n79766\t48103\tOdessa\tTX\tCrane County\tH1\n76943\t48105\tOzona\tTX\tCrockett County\tH1\n79370\t48107\tSpur\tTX\tCrosby County\tH1\n79322\t48107\tCrosbyton\tTX\tCrosby County\tH1\n79343\t48107\tLorenzo\tTX\tCrosby County\tH1\n79235\t48107\tFloydada\tTX\tCrosby County\tH1\n79243\t48107\tMcadoo\tTX\tCrosby County\tH1\n79357\t48107\tRalls\tTX\tCrosby County\tH1\n79847\t48109\tSalt flat\tTX\tCulberson County\tH1\n79855\t48109\tVan horn\tTX\tCulberson County\tH1\n79022\t48111\tDalhart\tTX\tDallam County\tH1\n79084\t48111\tStratford\tTX\tDallam County\tH1\n79087\t48111\tTexline\tTX\tDallam County\tH1\n79051\t48111\tKerrick\tTX\tDallam County\tH1\n75043\t48113\tGarland\tTX\tDallas County\tH1\n75098\t48113\tWylie\tTX\tDallas County\tH1\n75116\t48113\tDuncanville\tTX\tDallas County\tH1\n75146\t48113\tLancaster\tTX\tDallas County\tH1\n75106\t48113\tCedar hill\tTX\tDallas County\tH1\n75201\t48113\tDallas\tTX\tDallas County\tH1\n75216\t48113\tDallas\tTX\tDallas County\tH1\n75212\t48113\tDallas\tTX\tDallas County\tH1\n75234\t48113\tDallas\tTX\tDallas County\tH1\n75237\t48113\tDallas\tTX\tDallas County\tH1\n75227\t48113\tDallas\tTX\tDallas County\tH1\n75240\t48113\tDallas\tTX\tDallas County\tH1\n75244\t48113\tDallas\tTX\tDallas County\tH1\n75247\t48113\tDallas\tTX\tDallas County\tH1\n75251\t48113\tDallas\tTX\tDallas County\tH1\n75067\t48113\tLewisville\tTX\tDallas County\tH1\n75356\t48113\tDallas\tTX\tDallas County\tH1\n75357\t48113\tDallas\tTX\tDallas County\tH1\n75374\t48113\tDallas\tTX\tDallas County\tH1\n75242\t48113\tDallas\tTX\tDallas County\tH1\n75336\t48113\tDallas\tTX\tDallas County\tH1\n75342\t48113\tDallas\tTX\tDallas County\tH1\n75014\t48113\tIrving\tTX\tDallas County\tH1\n75039\t48113\tIrving\tTX\tDallas County\tH1\n75041\t48113\tGarland\tTX\tDallas County\tH1\n75159\t48113\tSeagoville\tTX\tDallas County\tH1\n75232\t48113\tDallas\tTX\tDallas County\tH1\n75220\t48113\tDallas\tTX\tDallas County\tH1\n75228\t48113\tDallas\tTX\tDallas County\tH1\n75062\t48113\tIrving\tTX\tDallas County\tH1\n75254\t48113\tDallas\tTX\tDallas County\tH1\n75001\t48113\tAddison\tTX\tDallas County\tH1\n76051\t48113\tGrapevine\tTX\tDallas County\tH1\n75390\t48113\tDallas\tTX\tDallas County\tH1\n75016\t48113\tIrving\tTX\tDallas County\tH1\n75354\t48113\tDallas\tTX\tDallas County\tH1\n75398\t48113\tDallas\tTX\tDallas County\tH1\n75040\t48113\tGarland\tTX\tDallas County\tH1\n75048\t48113\tSachse\tTX\tDallas County\tH1\n75137\t48113\tDuncanville\tTX\tDallas County\tH1\n75214\t48113\tDallas\tTX\tDallas County\tH1\n75231\t48113\tDallas\tTX\tDallas County\tH1\n75235\t48113\tDallas\tTX\tDallas County\tH1\n75238\t48113\tDallas\tTX\tDallas County\tH1\n75224\t48113\tDallas\tTX\tDallas County\tH1\n75243\t48113\tDallas\tTX\tDallas County\tH1\n75246\t48113\tDallas\tTX\tDallas County\tH1\n75060\t48113\tIrving\tTX\tDallas County\tH1\n75371\t48113\tDallas\tTX\tDallas County\tH1\n75315\t48113\tDallas\tTX\tDallas County\tH1\n75047\t48113\tGarland\tTX\tDallas County\tH1\n75019\t48113\tCoppell\tTX\tDallas County\tH1\n75050\t48113\tGrand prairie\tTX\tDallas County\tH1\n75051\t48113\tGrand prairie\tTX\tDallas County\tH1\n75049\t48113\tGarland\tTX\tDallas County\tH1\n75046\t48113\tGarland\tTX\tDallas County\tH1\n75088\t48113\tRowlett\tTX\tDallas County\tH1\n75202\t48113\tDallas\tTX\tDallas County\tH1\n75181\t48113\tMesquite\tTX\tDallas County\tH1\n75217\t48113\tDallas\tTX\tDallas County\tH1\n75230\t48113\tDallas\tTX\tDallas County\tH1\n75233\t48113\tDallas\tTX\tDallas County\tH1\n75236\t48113\tDallas\tTX\tDallas County\tH1\n75249\t48113\tDallas\tTX\tDallas County\tH1\n75241\t48113\tDallas\tTX\tDallas County\tH1\n75061\t48113\tIrving\tTX\tDallas County\tH1\n75080\t48113\tRichardson\tTX\tDallas County\tH1\n75287\t48113\tDallas\tTX\tDallas County\tH1\n75141\t48113\tHutchins\tTX\tDallas County\tH1\n75261\t48113\tDallas\tTX\tDallas County\tH1\n75360\t48113\tDallas\tTX\tDallas County\tH1\n75250\t48113\tDallas\tTX\tDallas County\tH1\n75099\t48113\tCoppell\tTX\tDallas County\tH1\n75089\t48113\tRowlett\tTX\tDallas County\tH1\n75115\t48113\tDesoto\tTX\tDallas County\tH1\n75134\t48113\tLancaster\tTX\tDallas County\tH1\n75138\t48113\tDuncanville\tTX\tDallas County\tH1\n75205\t48113\tDallas\tTX\tDallas County\tH1\n75211\t48113\tDallas\tTX\tDallas County\tH1\n75180\t48113\tBalch springs\tTX\tDallas County\tH1\n75215\t48113\tDallas\tTX\tDallas County\tH1\n75226\t48113\tDallas\tTX\tDallas County\tH1\n75225\t48113\tDallas\tTX\tDallas County\tH1\n75252\t48113\tDallas\tTX\tDallas County\tH1\n75253\t48113\tDallas\tTX\tDallas County\tH1\n75053\t48113\tGrand prairie\tTX\tDallas County\tH1\n75223\t48113\tDallas\tTX\tDallas County\tH1\n75085\t48113\tRichardson\tTX\tDallas County\tH1\n75355\t48113\tDallas\tTX\tDallas County\tH1\n75011\t48113\tCarrollton\tTX\tDallas County\tH1\n75378\t48113\tDallas\tTX\tDallas County\tH1\n75187\t48113\tMesquite\tTX\tDallas County\tH1\n75221\t48113\tDallas\tTX\tDallas County\tH1\n75044\t48113\tGarland\tTX\tDallas County\tH1\n75045\t48113\tGarland\tTX\tDallas County\tH1\n75123\t48113\tDesoto\tTX\tDallas County\tH1\n75149\t48113\tMesquite\tTX\tDallas County\tH1\n75203\t48113\tDallas\tTX\tDallas County\tH1\n75204\t48113\tDallas\tTX\tDallas County\tH1\n75208\t48113\tDallas\tTX\tDallas County\tH1\n75172\t48113\tWilmer\tTX\tDallas County\tH1\n75210\t48113\tDallas\tTX\tDallas County\tH1\n75339\t48113\tDallas\tTX\tDallas County\tH1\n75006\t48113\tCarrollton\t
